vi "round_2decimals.vi"(11 "Number":dbl) -> (3 "Rounded Number":dbl)   [LabVIEW 2018]
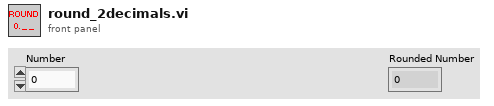
[diagram p1: front panel]
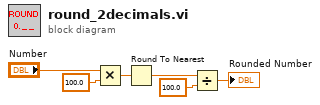
[diagram p0: block diagram]
diagram:
  n1 = Multiply(x="Number", y=100.0) -> (x*y=w4:dbl)
  n2 = Round To Nearest(number=w4) -> (nearest integer value=w3:dbl)
  n3 = Divide(x=w3, y=100.0) -> (x/y=→"Rounded Number":dbl)
